vi "MTM2_getSample_tangentActuatorAbsolutePositionSteps.vi"(8 "error in (no error)":errorcluster, 11 "tangentActuatorAbsolutePositionSteps_Ctl":T1) -> (0 "error out":errorcluster, 2 "function return":i32, 3 "tangentActuatorAbsolutePositionSteps_Ctl out":T1)   [LabVIEW 2018, in "SALLV_MTM2.lvlib"]
doc: "int MTM2_shm_getSample_tangentActuatorAbsolutePositionStepsLV(MTM2_tangentActuatorAbsolutePositionStepsLV *tangentActuatorAbsolutePositionSteps_Ctl );"
uses:
  SALLV_MTM2.lvlib
  DataTypes/tangentActuatorAbsolutePositionSteps.ctl
  SALLV_MTM2.so
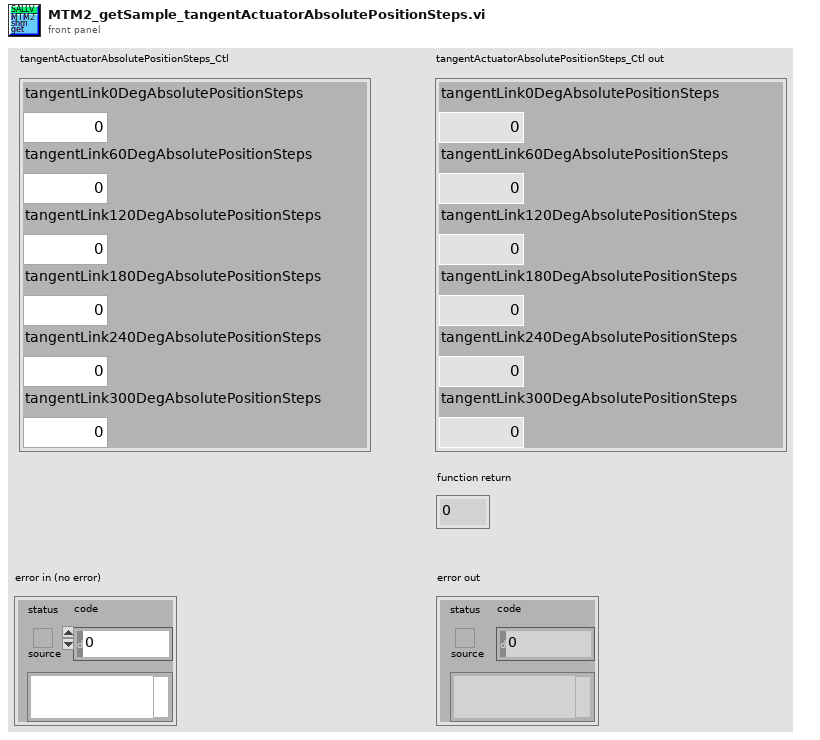
[diagram p1: front panel]
types:
  T1 = typedef "SALLV_MTM2.lvlib/tangentActuatorAbsolutePositionSteps.ctl" = cluster{"tangentLink0DegAbsolutePositionSteps":i32, "tangentLink60DegAbsolutePositionSteps":i32, "tangentLink120DegAbsolutePositionSteps":i32, "tangentLink180DegAbsolutePositionSteps":i32, "tangentLink240DegAbsolutePositionSteps":i32, "tangentLink300DegAbsolutePositionSteps":i32}
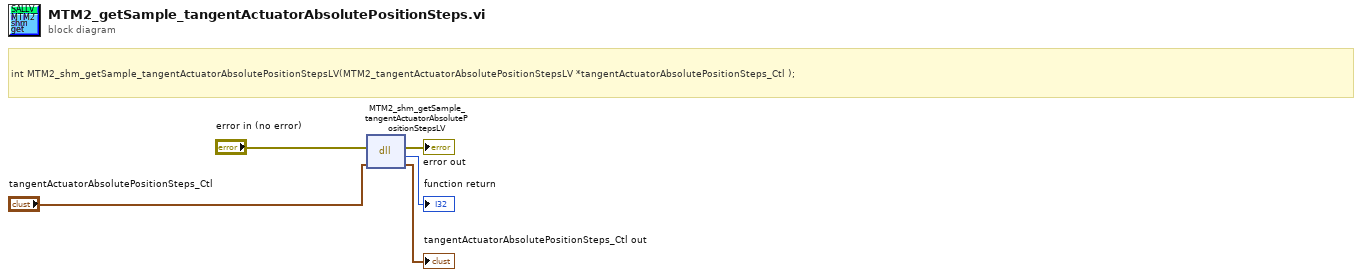
[diagram p0: block diagram]
diagram:
  # "int MTM2_shm_getSample_tangentActuatorAbsolutePositionStepsLV(MTM2_tangentActuatorAbsolutePositionStepsLV *tangentActuatorAbsolutePositionSteps_Ctl );"
  n1 = dll-call lib="home/ttsai/Document/salApiMTM2/SALLV_MTM2/SALLV_MTM2.*" fn="MTM2_shm_getSample_tangentActuatorAbsolutePositionStepsLV"(error in="error in (no error)", "tangentActuatorAbsolutePositionSteps_Ctl"="tangentActuatorAbsolutePositionSteps_Ctl") -> (error out=→"error out":errorcluster, →"function return":i32, "tangentActuatorAbsolutePositionSteps_Ctl"=→"tangentActuatorAbsolutePositionSteps_Ctl out":T1)  [unwired: 2 in, 1 out]
